vi "ETAB_decodeur.vi"(0 "chaine entree":string) -> (1 "Args":string[](array[string]), 2 "nb args":u16, 3 "OK done":bool)   [LabVIEW 2011]
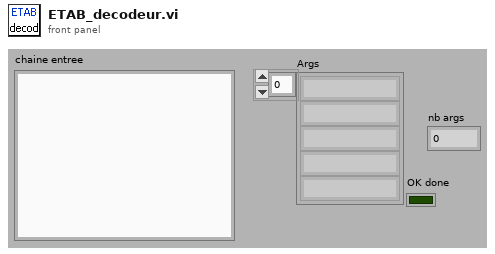
[diagram p1: front panel]
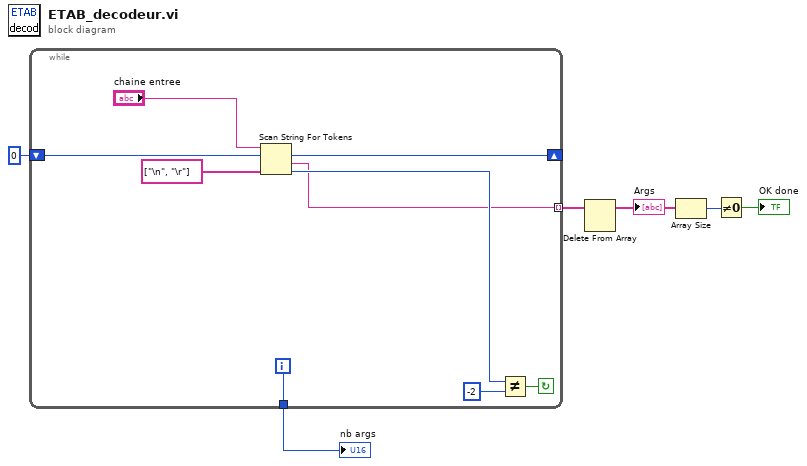
[diagram p0: block diagram]
diagram:
  n1 = while {
    shift-right: [w8] -> _
    shift-left: 0 ("offset past token") -> [w11]
    tunnel: [w10] -> w1
    tunnel: [w7] -> w5 mode=indexing
    i -> [w10]
    stop <- w14 continue-if-true
    n2 = Scan String For Tokens(6:string[] ["\n", "\r"] ("delimiters (\\s,\\t,\\r,\\n)"), 8:w11, 9:"chaine entree") -> (0:w12:i32, 1:w7:string, 2:w8:i32)  [unwired: 3 in, 1 out]
    n3 = Not Equal?(x=w12, y=-2) -> (x != y?=w14:bool)
  }
  "nb args" <- w1
  n4 = Delete From Array(array=w5) -> (array with subset deleted=w4:string[])  [unwired: 2 in, 1 out]
  "Args" <- w4
  n5 = Array Size(array=w4) -> (size(s)=w3:i32)
  n6 = Not Equal To 0?(x=w3) -> (x != 0?=→"OK done":bool)
